vi "H036 Harsh Pandit SCADA Lab 6a Sem 6.vi"() -> ()   [LabVIEW 2018]
panel:
  out "Reverse Array":dbl[](array[numeric])
  out "Array":dbl[](array[numeric])
  # "Experiment 6a: Create one dimensional numeric array of 7 elements using random numbers.\nAlso obtain reverse of the array"
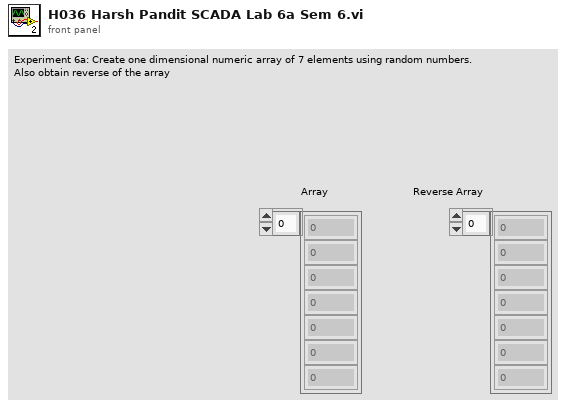
[diagram p1: front panel]
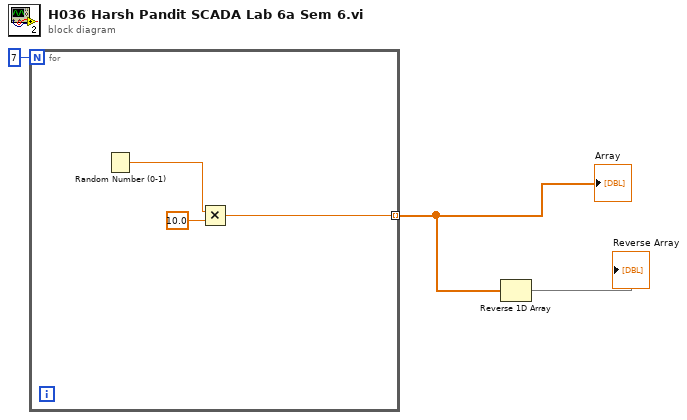
[diagram p0: block diagram]
diagram:
  n1 = for {
    N: 7 -> [_]
    tunnel: [w4] -> w2 mode=indexing
    n2 = Random Number (0-1)() -> (number: 0 to 1=w6:dbl)
    n3 = Multiply(x=w6, y=10.0) -> (x*y=w4:dbl)
  }
  "Array" <- w2
  n4 = Reverse 1D Array(array=w2) -> (reversed array=→"Reverse Array":dbl[])
